vi "Labview offline.vi"() -> ()   [LabVIEW 2019]
uses:
  <vilib>/sound2/lvsound2.llb/Sampling Mode.ctl
  <vilib>/sound2/lvsound2.llb/Sound File Position.ctl
  <vilib>/sound2/lvsound2.llb/Sound File Read Open.vi
  <vilib>/sound2/lvsound2.llb/Sound File Info (refnum).vi
  <vilib>/sound2/lvsound2.llb/Sound File Read (DBL).vi
  <vilib>/sound2/lvsound2.llb/Sound Output Write (DBL).vi
  <vilib>/Analysis/NI_AAL_SigProc.lvlib
  <vilib>/gmath/NI_Gmath.lvlib
panel:
  out "Envelope do Sinal":dynamicdata(graph)
  out "Ritmo Cardíaco Médio":dbl format="%0.2f"
  in  "Medição":bool
  out "Taquicardia":bool
  out "Ritmo Cardíaco Normal":bool
  out "Bradicardia":bool
  in  "Continuar":bool
  out "Sinal Amplificado":waveform(dbl)[](graph)
  out "Sinal Amplificado e Filtrado":dynamicdata(graph)
  in  "Pulmões  ou Coração (pressionar botão)":bool
  out "Número total de Amostras/canal":u32
  out "Taxa de Amostragem do Ficheiro (S/s))":dbl
  in  "Path - Ficheiro Som Cardíaco":path
  in  "Controlador de Threshold":dbl(slide) scale=0.0..0.01
  out "Ritmo Cardíaco Instantaneo":dbl
  in  "Terminar Medições":bool
  out "Offline Sound":dbl[](array[numeric])
  # "Estetoscópio Digital"
  # "Resultados"
  # "Configurações e Controlos"
  # "Parâmetros do Ficheiro de Som"
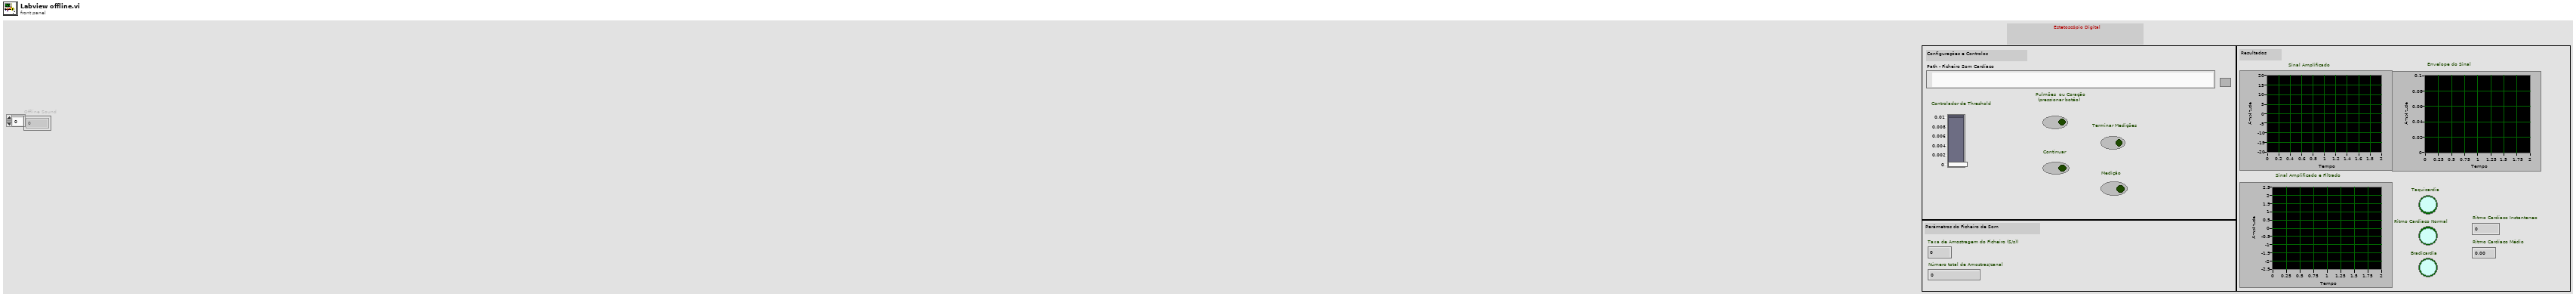
[diagram p1: front panel]
types:
  T1 = typedef "Sampling Mode.ctl" = i32
  T2 = typedef "Sound File Refnum.ctl" = refnum<file>
  T3 = typedef "Sound Data Format.ctl" = cluster{"sample rate (S/s)":dbl, "number of channels":i32, "bits per sample":i32}
  T4 = typedef "Sound Output Task ID.ctl" = u32
  T5 = typedef "Sound File Position.ctl" = u16
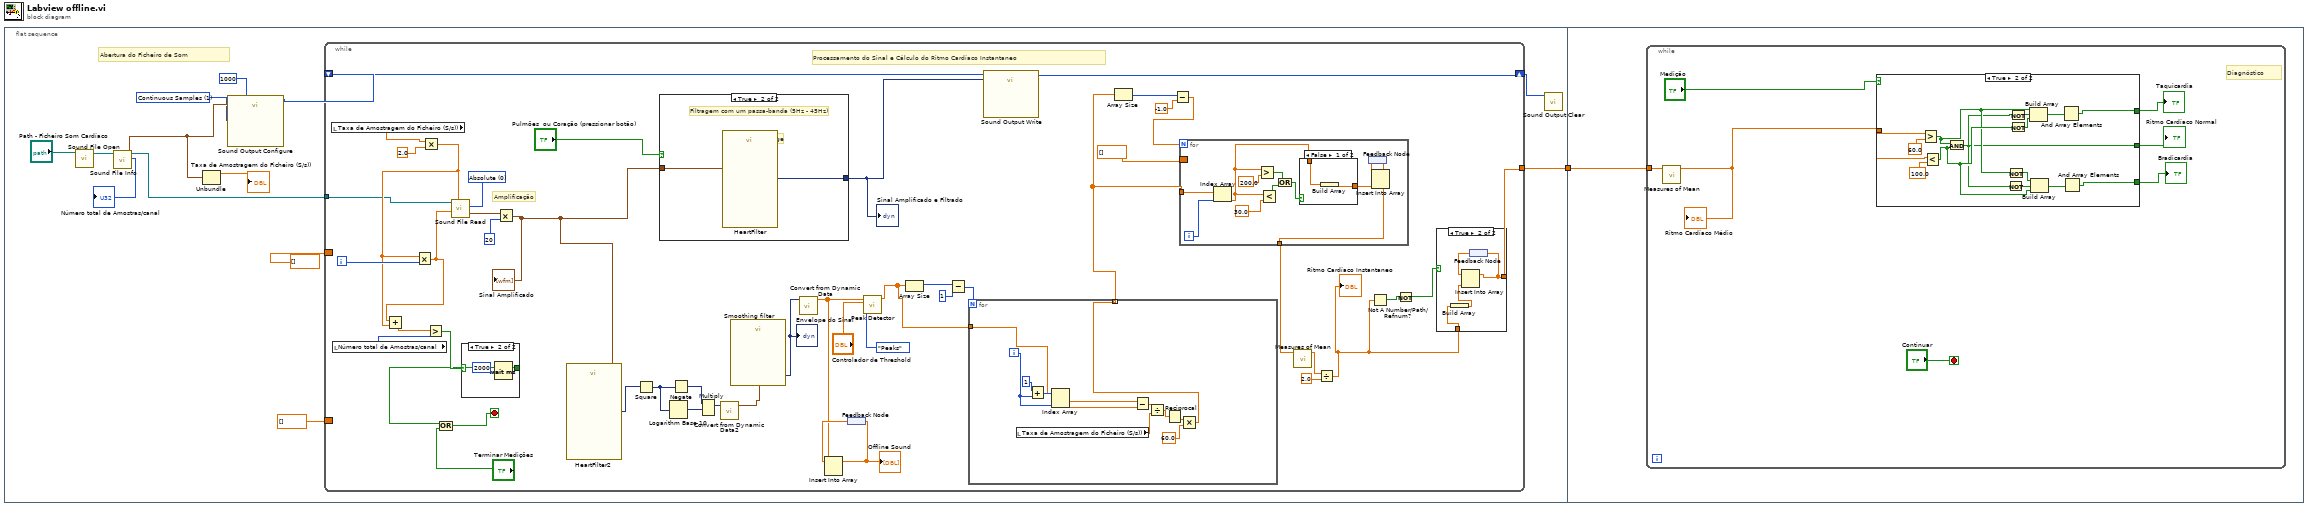
[diagram p0: block diagram]
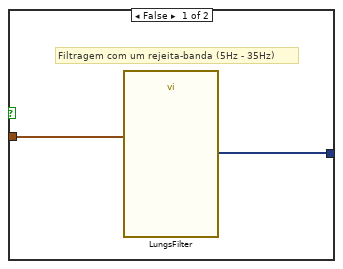
[diagram p5: hidden frame]
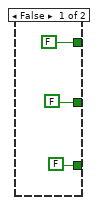
[diagram p6: hidden frame]
diagram:
  n1 = flat-sequence {
    tunnel: [w2] -> w1
    tunnel: w1 -> [w99]
    frame #0 {
      w3 = T1 1 items=["Finite Samples", "Continuous Samples"] ("sample mode")
      # "Abertura do Ficheiro de Som"
      n2 = call-poly <vilib>:"Sound File Open.vi"("path"="Path - Ficheiro Som Cardíaco") -> ("sound file refnum"=w6:T2)  [unwired: 9 in, 1 out]
      n3 = call-poly <vilib>:"Sound File Info.vi"("sound file refnum"=w6) -> ("sound format"=w8:T3, "total number of samples/ch"=→"Número total de Amostras/canal":u32, "sound file refnum out"=w11:T2)  [unwired: 7 in, 1 out]
      n4 = Unbundle(w8) -> ("sample rate (S/s)"=→"Taxa de Amostragem do Ficheiro (S/s))":dbl)  [unwired: 2 out]
      n5 = call <vilib>:"Sound Output Configure.vi"("number of samples/ch"=1000, "sample mode"=w3, "sound format"=w8) -> ("task ID"=w10:T4)  [unwired: 3 in, 5 out]
      n6 = while {
        shift-right: [w61] -> w12
        shift-left: w10 -> [w59]
        tunnel: [w39] -> w2
        border: dbl[] [] -> [_]
        border: dbl[] [] -> [_]
        tunnel: w11 -> [w24]
        i -> [w55]
        stop <- w34 stop-if-true
        w60 = T5 0 items=["Absolute"=0, "Relative"=2] ("position mode")
        # "Processamento do Sinal e Cálculo do Ritmo Cardíaco Instantaneo"
        # "Filter Stage"
        # "Amplificação"
        n7 = local read "Taxa de Amostragem do Ficheiro (S/s))"() -> (w53:dbl)
        n8 = local read "Número total de Amostras/canal"() -> (w43:u32)
        n9 = Multiply(x=w53, y=2.0) -> (x*y=w42:dbl)
        n10 = Multiply(x=w42, y=w55) -> (x*y=w58:dbl)
        n11 = Add(x=w58, y=w42) -> (x+y=w57:dbl)
        n12 = Greater?(x=w57, y=w43) -> (0:w56:bool)
        n13 = call-poly <vilib>:"Sound File Read.vi"("number of samples/ch (-1: all)"=w42, "position offset"=w58, "position mode"=w60, "sound file refnum"=w24) -> ("data"=w32:waveform(dbl)[])  [unwired: 3 in, 4 out]
        n14 = case shown="True" w56 {
          selector: w56 -> [w92 w94]
          tunnel: [w92 w94] -> w36
          frame False {
          }
          frame True {
            n15 = Wait (ms)(milliseconds to wait=u32 2000) -> ()  [unwired: 1 out]
          }
        }
        n16 = Compound Arithmetic op=OR(w36, "Terminar Medições") -> (w34:bool)
        n17 = Multiply(x=w32, y=20) -> (x*y=w21:waveform(dbl)[])
        "Sinal Amplificado" <- w21
        n18 = call "HeartFilter2"("Signal"=w21) -> ("Filtered Signal"=w22:dynamicdata)  [unwired: 9 in, 1 out]
        n19 = Square(x=w22) -> (x^2=w29:dynamicdata)
        n20 = case shown="True" "Pulmões  ou Coração (pressionar botão)" {
          tunnel: w21 -> [w96 w98]
          tunnel: [w95 w97] -> w25
          frame False {
            # "Filtragem com um rejeita-banda (5Hz - 35Hz)"
            n21 = call "LungsFilter"("Signal"=w96) -> ("Filtered Signal"=w95:dynamicdata)  [unwired: 9 in, 1 out]
          }
          frame True {
            # "Filtragem com um passa-banda (5Hz - 45Hz)"
            n22 = call "HeartFilter"("Signal"=w98) -> ("Filtered Signal"=w97:dynamicdata)  [unwired: 9 in, 1 out]
          }
        }
        "Sinal Amplificado e Filtrado" <- w25
        n23 = Logarithm Base 10(1:w29) -> (0:w31:dynamicdata)
        n24 = Negate(x=w29) -> (-x=w30:dynamicdata)
        n25 = Multiply(1:w31, 2:w30) -> (0:w28:dynamicdata)  [unwired: 1 in, 1 out]
        n26 = call "Convert from Dynamic Data2"("Dynamic Data Type"=w28) -> ("Waveform"=w15:waveform(dbl))  [unwired: 3 in]
        n27 = call "Smoothing filter"("Signal"=w15) -> ("Filtered Signal"=w16:dynamicdata)  [unwired: 9 in, 1 out]
        "Envelope do Sinal" <- w16
        n28 = call "Convert from Dynamic Data"("Dynamic Data Type"=w16) -> ("Array"=w23:dbl[])  [unwired: 3 in]
        n29 = feedback #1() -> (w33:dbl[])
        n30 = Insert Into Array(array=w33, new element=w23) -> (w27:dbl[])  [unwired: 1 in]
        "Offline Sound" <- w27
        n31 = feedback-in #1(w27) -> ()
        n32 = call <vilib>:"Peak Detector.vi"("peaks/valleys"=enum32{"Peaks", "Valleys"}."Peaks", "threshold"="Controlador de Threshold", "X"=w23) -> ("Locations"=w20:dbl[])  [unwired: 4 in, 4 out]
        n33 = Array Size(array=w20) -> (size(s)=w48:i32)
        n34 = Subtract(x=w48, y=1) -> (x-y=w49:i32)
        n35 = for {
          N: w49 -> [_]
          tunnel: w20 -> [w82]
          tunnel: [w81] -> w41 mode=indexing
          i -> [w80]
          n36 = local read "Taxa de Amostragem do Ficheiro (S/s))"() -> (w89:dbl)
          n37 = Add(x=1, y=w80) -> (x+y=w85:i32)
          n38 = Index Array(array=w82, index #1=w85, index #2=w80) -> (element #1=w86:dbl, element #2=w87:dbl)
          n39 = Subtract(x=w86, y=w87) -> (x-y=w88:dbl)
          n40 = Divide(x=w88, y=w89) -> (x/y=w90:dbl)
          n41 = Reciprocal(x=w90) -> (1/x=w91:dbl)
          n42 = Multiply(x=w91, y=60.0) -> (x*y=w81:dbl)
        }
        n43 = call-poly <vilib>:"Sound Output Write.vi"("data"=w25, "task ID"=w59) -> ("task ID out"=w61:T4)  [unwired: 2 in, 7 out]
        n44 = Array Size(array=w41) -> (size(s)=w46:i32)
        n45 = Subtract(x=w46, y=-1.0) -> (x-y=w45:dbl)
        n46 = for {
          N: w45 -> [_]
          tunnel: w41 -> [w71]
          tunnel: [w67] -> w40
          border: dbl[] [] -> [_]
          i -> [w72]
          n47 = Index Array(array=w71, index=w72) -> (element=w70:dbl)
          n48 = Greater?(x=w70, y=200.0) -> (0:w75:bool)
          n49 = Less?(x=w70, y=30.0) -> (x < y?=w74:bool)
          n50 = Or(x=w75, y=w74) -> (x .or. y?=w73:bool)
          n51 = case shown="False" w73 {
            tunnel: w70 -> [w79 _]
            tunnel: [w78 _] -> w69
            frame False {
              n52 = Build Array(w79) -> (w78:dbl[])
            }
            frame True {
            }
          }
          n53 = feedback #2() -> (w68:dbl[])
          n54 = Insert Into Array(array=w68, new element=w69) -> (w67:dbl[])  [unwired: 1 in]
          n55 = feedback-in #2(w67) -> ()
        }
        n56 = call <vilib>:"Measures of Mean.vi"("x array"=w40) -> ("mean value"=w18:dbl)  [unwired: 9 in, 1 out]
        n57 = Divide(x=w18, y=2.0) -> (x/y=w19:dbl)
        "Ritmo Cardíaco Instantaneo" <- w19
        n58 = Not A Number/Path/Refnum?(number/path/refnum=w19) -> (NaN/Path/Refnum?=w38:bool)
        n59 = Not(x=w38) -> (.not. x?=w37:bool)
        n60 = case shown="True" w37 {
          tunnel: [_ w65] -> w39
          tunnel: w19 -> [_ w64]
          frame False {
          }
          frame True {
            n61 = Build Array(w64) -> (w63:dbl[])
            n62 = feedback #3() -> (w66:dbl[])
            n63 = Insert Into Array(array=w66, new element=w63) -> (w65:dbl[])  [unwired: 1 in]
            n64 = feedback-in #3(w65) -> ()
          }
        }
      }
      n65 = call <vilib>:"Sound Output Clear.vi"("task ID"=w12) -> ()  [unwired: 10 in, 1 out]
    }
    frame #1 {
      n66 = while {
        tunnel: w99 -> [w103]
        stop <- "Continuar" stop-if-true
        # "Diagnóstico"
        n67 = call <vilib>:"Measures of Mean.vi"("x array"=w103) -> ("mean value"=w101:dbl)  [unwired: 9 in, 1 out]
        "Ritmo Cardíaco Médio" <- w101
        n68 = case shown="True" "Medição" {
          tunnel: w101 -> [_ w121]
          tunnel: [FALSE w112] -> w106
          tunnel: [FALSE w111] -> w105
          tunnel: [FALSE w110] -> w104
          frame False {
          }
          frame True {
            n69 = Greater?(x=w121, y=60.0) -> (0:w114:bool)
            n70 = Less?(x=w121, y=100.0) -> (x < y?=w116:bool)
            n71 = And(x=w114, y=w116) -> (x .and. y?=w111:bool)
            n72 = Not(x=w111) -> (.not. x?=w117:bool)
            n73 = Not(x=w114) -> (.not. x?=w115:bool)
            n74 = Not(x=w111) -> (.not. x?=w119:bool)
            n75 = Not(x=w116) -> (.not. x?=w118:bool)
            n76 = Build Array(w114, w119, w118) -> (w120:bool[])
            n77 = Build Array(w115, w117, w116) -> (w113:bool[])
            n78 = And Array Elements(Boolean array=w120) -> (logical AND=w110:bool)
            n79 = And Array Elements(Boolean array=w113) -> (logical AND=w112:bool)
          }
        }
        "Taquicardia" <- w104
        "Ritmo Cardíaco Normal" <- w105
        "Bradicardia" <- w106
      }
    }
  }
